vi "RollN.vi"() -> ()   [LabVIEW 2014]
panel:
  out "Complete Roll History":i32[](array[numeric])
  out "Roll Value History":i32[](graph)
  in  "Roll N Times":i32=50
  in  "Die N Sides":i32=6
  out "Roll Number":i32
  # "Roll a virtual die N times"
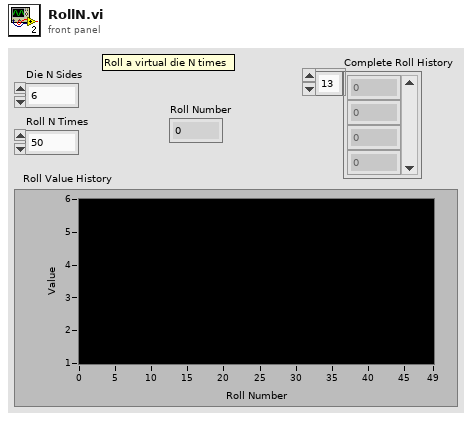
[diagram p1: front panel]
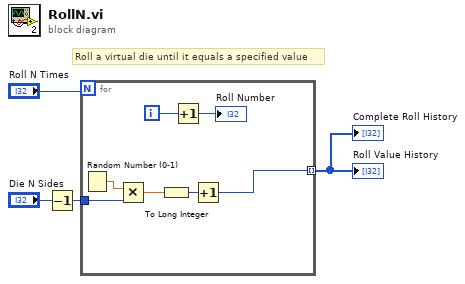
[diagram p0: block diagram]
diagram:
  # "Roll a virtual die until it equals a specified value"
  n1 = Decrement(x="Die N Sides") -> (x-1=w1:i32)
  n2 = for {
    N: "Roll N Times" -> [_]
    tunnel: [w8] -> w2 mode=indexing
    tunnel: w1 -> [w5]
    i -> [w7]
    n3 = Random Number (0-1)() -> (number: 0 to 1=w11:dbl)
    n4 = Multiply(x=w11, y=w5) -> (x*y=w10:dbl)
    n5 = To Long Integer(number=w10) -> (32bit integer=w9:i32)
    n6 = Increment(x=w7) -> (x+1=→"Roll Number":i32)
    n7 = Increment(x=w9) -> (x+1=w8:i32)
  }
  "Roll Value History" <- w2
  "Complete Roll History" <- w2
